vi "addElf.vi"(8 "error in (no error)":errorcluster, 10 "Elf.lvclass":refnum<class "Elf.lvclass">, 11 "ElfHeap in":refnum<class "ElfHeap.lvclass">) -> (0 "error out":errorcluster, 3 "ElfHeap out":refnum<class "ElfHeap.lvclass">)   [LabVIEW 2017, in "ElfHeap.lvclass"]
uses:
  ElfHeap.lvclass
  Elf/Elf.lvclass
  ElfHeap.lvclass/ElfHeap.ctl
  Elf/Elf.lvclass/Elf.ctl
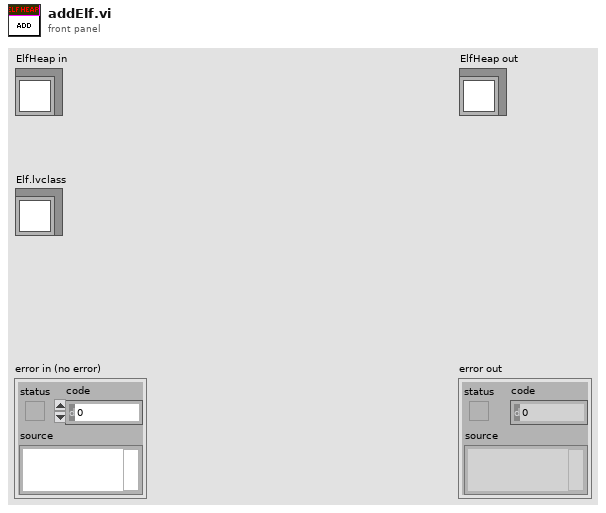
[diagram p1: front panel]
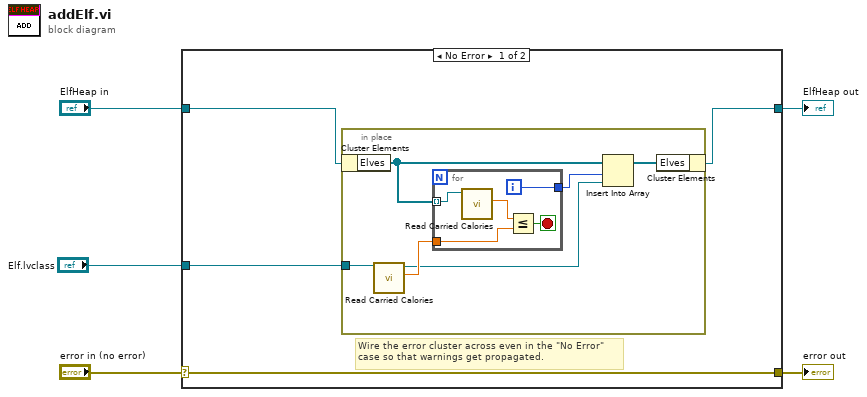
[diagram p0: block diagram]
diagram:
  n1 = case shown="No Error" "error in (no error)" {
    selector: "error in (no error)" -> [w9 w22]
    tunnel: [w9 w22] -> w4
    tunnel: [w6 w21] -> w2
    tunnel: "ElfHeap in" -> [w8 w21]
    tunnel: "Elf.lvclass" -> [w7 _]
    frame No Error {
      # "Wire the error cluster across even in the \"No Error\"\ncase so that warnings get propagated."
      n2 = in-place {
        in-place-border: w7 -> [w15]
        n3 = in-place-cluster #1(w8) -> ("Elves"=w13:refnum<class "Elf.lvclass">[])
        n4 = call "Read Carried Calories.vi"("Elf in"=w15) -> ("Carried Calories"=w14:dbl, "Elf out"=w12:refnum<class "Elf.lvclass">)  [unwired: 8 in, 1 out]
        n5 = for {
          tunnel: w13 -> [w20] mode=indexing
          tunnel: w14 -> [w18]
          tunnel: [w16] -> w11
          i -> [w16]
          stop <- w17 stop-if-true
          n6 = call "Read Carried Calories.vi"("Elf in"=w20) -> ("Carried Calories"=w19:dbl)  [unwired: 8 in, 2 out]
          n7 = Less Or Equal?(x=w19, y=w18) -> (x <= y?=w17:bool)
        }
        n8 = Insert Into Array(array=w13, index=w11, new element=w12) -> (w10:refnum<class "Elf.lvclass">[])
        n9 = in-place-cluster #1("Elves"=w10) -> (w6:refnum<class "ElfHeap.lvclass">)
      }
    }
    frame Error {
    }
  }
  "error out" <- w4
  "ElfHeap out" <- w2
